vi "Process Name.vi"(11 "Process Name":string) -> (3 "Process Name":string="_Main")   [LabVIEW 2020, in "Main_Process.lvlib" / "Internal Messaging Library.lvlib"]
doc: "Appends a suffix to the Name so that there is at least one bit of string for creating a queue name.\n\n2/2025 Erich Schlieper"
uses:
  Internal Messaging Library.lvlib
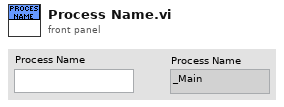
[diagram p1: front panel]
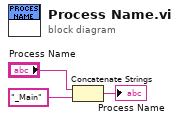
[diagram p0: block diagram]
diagram:
  n1 = Concatenate Strings("Process Name", "_Main") -> (→"Process Name":string)
